vi "Read Session.vi"(8 "Error In":errorcluster, 11 "Listener In":refnum<class "Listener.lvclass">) -> (0 "Error Out":errorcluster, 2 "Session":refnum<class "Session.lvclass">, 3 "Listener Out":refnum<class "Listener.lvclass">)   [LabVIEW 2021, in "Field_RnD_Services_LIBSSH2_Toolkit.lvlib" / "Listener.lvclass"]
doc: "Gets the Session object used to create this Listener object."
uses:
  Listener.lvclass
  Session/Session.lvclass
  Listener.lvclass/Listener.ctl
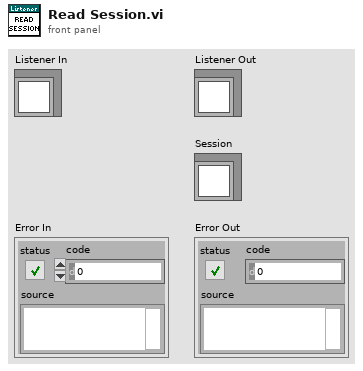
[diagram p1: front panel]
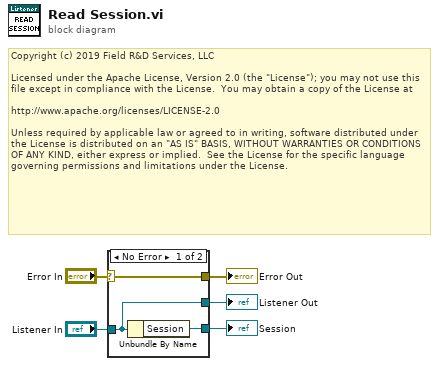
[diagram p0: block diagram]
diagram:
  # "Copyright (c) 2019 Field R&D Services, LLC\n\nLicensed under the Apache License, Version 2.0 (the \"License\"); you may not use this file except in compliance with the License.  You may obtain a copy of the License at\n\nhttp://www.apache.org/licenses/LICENSE-2.0\n\nUnless required by applicable law or agreed to in writing, software distributed under the License is distributed on an \"AS IS\" BASIS, WITHOUT WARRANTIES OR CONDITIONS OF ANY KIND, either express or implied.  See the License for the specific language governing permissions and limitations under the License."
  n1 = case shown="No Error" "Error In" {
    selector: "Error In" -> [w7 w10]
    tunnel: "Listener In" -> [w8 w9]
    tunnel: [w8 w9] -> w2
    tunnel: [w7 w10] -> w4
    tunnel: [w6 _] -> w1
    frame No Error {
      n2 = Unbundle By Name(w8) -> ("Session"=w6:refnum<class "Session.lvclass">)
    }
    frame Error {
    }
  }
  "Error Out" <- w4
  "Listener Out" <- w2
  "Session" <- w1
